vi "Read DC power voltage and current.vi"(8 "error in (no error)":errorcluster, 10 "Channel Select":enum16{"Channel 1", "Channel 2", "Channel 3"}(ring), 11 "DC power COM":refnum<visa-resource-name>) -> (0 "error out":errorcluster, 1 "Current (mA)":dbl, 2 "Voltage (V)":dbl, 3 "DC power COM out":refnum<visa-resource-name>)   [LabVIEW 2017]
uses:
  <instrlib>/Keithley KE22xx Series/Keithley KE22xx Series.lvlib
panel:
  out "Current":string
  out "Voltage":string
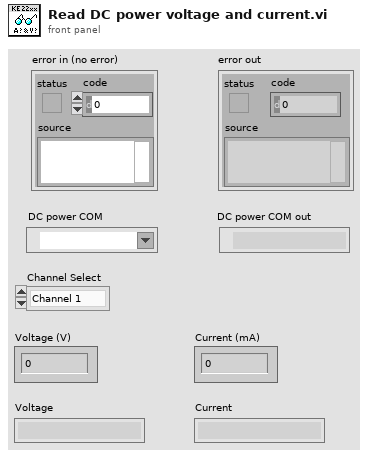
[diagram p1: front panel]
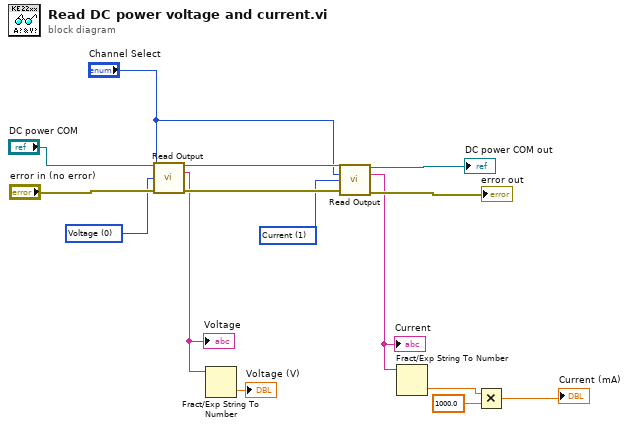
[diagram p0: block diagram]
diagram:
  w8 = u16 0 items=["Voltage", "Current", "Power"] ("Measurement Function (0:Voltage)")
  w9 = u16 1 items=["Voltage", "Current", "Power"] ("Measurement Function (0:Voltage)")
  n1 = call <instrlib>:"Read Output.vi"("VISA resource name"="DC power COM", "Channel Select"="Channel Select", "Measurement Function (0:Voltage)"=w8, "error in (no error)"="error in (no error)") -> ("VISA resource name out"=w15:refnum<visa-resource-name>, "Measurement"=w7:string, "error out"=w14:errorcluster)  [unwired: 9 in]
  "Voltage" <- w7
  n2 = Fract/Exp String To Number(string=w7) -> (number=→"Voltage (V)":dbl)  [unwired: 3 in, 1 out]
  n3 = call <instrlib>:"Read Output.vi"("VISA resource name"=w15, "Channel Select"="Channel Select", "Measurement Function (0:Voltage)"=w9, "error in (no error)"=w14) -> ("VISA resource name out"=→"DC power COM out":refnum<visa-resource-name>, "Measurement"=w4:string, "error out"=→"error out":errorcluster)  [unwired: 9 in]
  "Current" <- w4
  n4 = Fract/Exp String To Number(string=w4) -> (number=w2:dbl)  [unwired: 3 in, 1 out]
  n5 = Multiply(x=w2, y=1000.0) -> (x*y=→"Current (mA)":dbl)
